vi "UG-DGXMLGen.vi"() -> ()   [LabVIEW 2012]
uses:
  <vilib>/xml/Load XML File.vi
  <vilib>/xml/Close Reference(Node).vi
  <resource>/objmgr/DOMUserDefRef.rc
  <vilib>/xml/NI_XML.lvlib
panel:
  out "error out":errorcluster
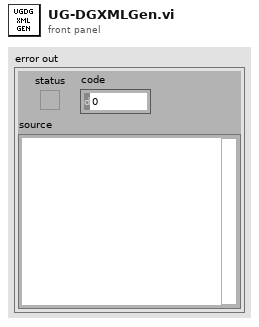
[diagram p1: front panel]
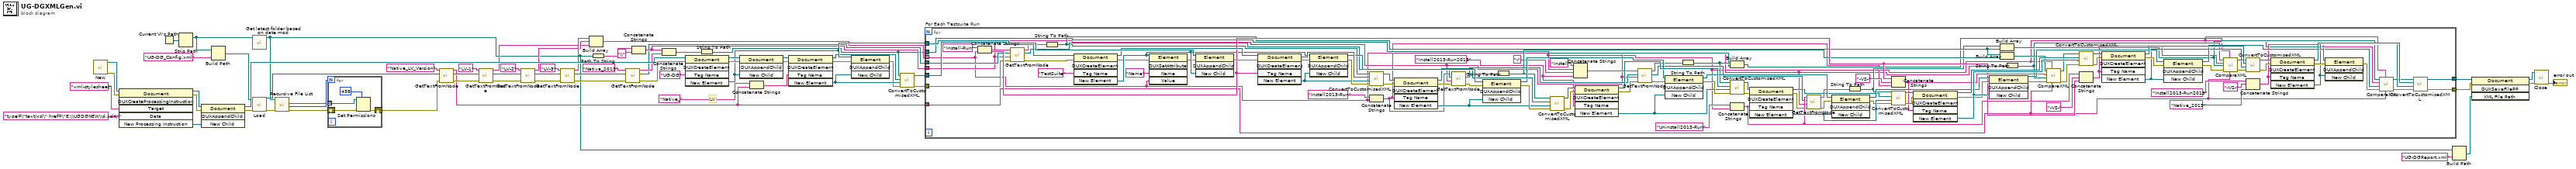
[diagram p0: block diagram]
diagram:
  # "LV"
  n1 = call <vilib>:"New.vi"() -> ("error out"=w59:errorcluster, "DOM document out"=w60:refnum<k20>)  [unwired: 1 in, 7 out]
  n2 = invoke class="Document" method="DUXCreateProcessingInstruction"(reference=w60, error in=w59, "Target"="xml-stylesheet" ("Value"), "Data"="type=\"text/xsl\" href=\"E:\\UGDGNEW\\d.xslt\"") -> (reference out=w65:refnum<k20>, error out=w64:errorcluster, "New Processing Instruction"=w63:refnum<k20>)  [unwired: 2 in, 3 out]
  n3 = Current VI's Path() -> (path=w8:path)
  n4 = Strip Path(path=w8) -> (stripped path=w7:path)  [unwired: 1 out]
  n5 = invoke class="Document" method="DUXAppendChild"(reference=w65, error in=w64, "New Child"=w63) -> (reference out=w58:refnum<k20>, error out=w27:errorcluster)  [unwired: 1 in, 2 out]
  n6 = Build Path(base path=w7, name or relative path="UG-DG_Config.xml") -> (appended path=w15:path)
  n7 = call "Get latest folder based on date mod.vi"("path"=w7) -> ("appended path"=w6:path)  [unwired: 10 in]
  n8 = call-poly <vilib>:"Load.vi"("path to XML document"=w15, "error in (no error)"=w27) -> ("DOM document out"=w42:refnum<k20>, "error out"=w2:errorcluster)  [unwired: 11 in, 1 out]
  n9 = call <vilib>:"Recursive File List.vi"("error in (no error)"=w2, "Folder Path"=w6) -> ("error out"=w3:errorcluster, "Number of Files"=w5:i32, "All Files in Dir"=w4:path[])  [unwired: 5 in, 2 out]
  n10 = for {
    N: w5 -> [_]
    tunnel: w4 -> [w71] mode=indexing
    shift-right: [w69] -> w1
    shift-left: w3 -> [w68]
    n11 = Set Permissions(7:i16 438 ("permissions"), 8:w68, 11:w71) -> (0:w69:errorcluster)  [unwired: 2 in, 1 out]
  }
  n12 = call "GetTextFromNode.vi"("error in (no error)"=w1, "node in"=w42, "Text"="Native_LV_Version" ("XPath expression")) -> ("error out"=w33:errorcluster, "node out"=w40:refnum<k20>, "Failure-db path"=w9:string)  [unwired: 6 in]
  n13 = call "GetTextFromNode.vi"("error in (no error)"=w33, "node in"=w40, "Text"="LV-1") -> ("error out"=w34:errorcluster, "node out"=w36:refnum<k20>, "Failure-db path"=w30:string)  [unwired: 6 in]
  n14 = call "GetTextFromNode.vi"("error in (no error)"=w34, "node in"=w36, "Text"="LV-2") -> ("error out"=w28:errorcluster, "node out"=w35:refnum<k20>, "Failure-db path"=w31:string)  [unwired: 6 in]
  n15 = call "GetTextFromNode.vi"("error in (no error)"=w28, "node in"=w35, "Text"="LV-3") -> ("error out"=w11:errorcluster, "node out"=w12:refnum<k20>, "Failure-db path"=w32:string)  [unwired: 6 in]
  n16 = Build Array(w32, w31, w30) -> (w29:string[])
  n17 = Path To String(path=w6) -> (string=w10:string)
  n18 = call "GetTextFromNode.vi"("error in (no error)"=w11, "node in"=w12, "Text"="Native_2013") -> ("error out"=w25:errorcluster, "node out"=w20:refnum<k20>, "Failure-db path"=w23:string)  [unwired: 6 in]
  n19 = Concatenate Strings(w10, "\\" ("string")) -> (w21:string)
  n20 = Concatenate Strings(w21, w23) -> (w22:string)
  n21 = invoke class="Document" method="DUXCreateElement"(reference=w58, error in=w25, "Tag Name"="UG-DG") -> (reference out=w66:refnum<k20>, error out=w57:errorcluster, "New Element"=w56:refnum<k20>)  [unwired: 2 in, 2 out]
  n22 = String To Path(string=w22) -> (path=w19:path)
  n23 = invoke class="Document" method="DUXAppendChild"(reference=w66, error in=w57, "New Child"=w56) -> (reference out=w54:refnum<k20>, error out=w55:errorcluster)  [unwired: 1 in, 2 out]
  n24 = Concatenate Strings("Native_" ("Tag Name"), w9) -> (w43:string)
  n25 = invoke class="Document" method="DUXCreateElement"(reference=w54, error in=w55, "Tag Name"=w43) -> (reference out=w51:refnum<k20>, error out=w53:errorcluster, "New Element"=w52:refnum<k20>)  [unwired: 2 in, 2 out]
  n26 = invoke class="Element" method="DUXAppendChild"(reference=w56, error in=w53, "New Child"=w52) -> (error out=w50:errorcluster)  [unwired: 1 in, 3 out]
  n27 = call "ConvertToCustomisedXML.vi"("error in"=w50, "New Element"=w52, "DOM document"=w51, "Path"=w19) -> ("error out"=w18:errorcluster, "DOM document out"=w17:refnum<k20>)  [unwired: 6 in]
  n28 = for "For Each Testsuite Run" {
    tunnel: w56 -> [w176]
    tunnel: w29 -> [w72] mode=indexing
    tunnel: [w118] -> w49
    tunnel: w17 -> [w177]
    tunnel: [w113] -> w45
    tunnel: w20 -> [w111]
    tunnel: w18 -> [w110]
    tunnel: w21 -> [w75]
    tunnel: w19 -> [w87]
    tunnel: w9 -> [w73]
    w76 = "Install2013-Run2013"
    n29 = Concatenate Strings("Install-Run", w72) -> (w112:string)
    n30 = call "GetTextFromNode.vi"("error in (no error)"=w110, "Failure db-folderpath"=w75, "node in"=w111, "Text"=w112) -> ("error out"=w109:errorcluster, "node out"=w106:refnum<k20>, "Failure-db path"=w103:string)  [unwired: 5 in]
    n31 = String To Path(string=w103) -> (path=w91:path)
    n32 = invoke class="Document" method="DUXCreateElement"(reference=w177, error in=w109, "Tag Name"="TestSuite") -> (reference out=w174:refnum<k20>, error out=w82:errorcluster, "New Element"=w83:refnum<k20>)  [unwired: 2 in, 2 out]
    n33 = invoke class="Element" method="DUXSetAttribute"(reference=w83, error in=w82, "Name"="Name", "Value"=w72) -> (error out=w81:errorcluster)  [unwired: 1 in, 4 out]
    n34 = invoke class="Element" method="DUXAppendChild"(reference=w176, error in=w81, "New Child"=w83) -> (error out=w122:errorcluster)  [unwired: 1 in, 3 out]
    n35 = invoke class="Document" method="DUXCreateElement"(reference=w174, error in=w122, "Tag Name"=w112) -> (reference out=w173:refnum<k20>, error out=w171:errorcluster, "New Element"=w155:refnum<k20>)  [unwired: 2 in, 2 out]
    n36 = invoke class="Element" method="DUXAppendChild"(reference=w83, error in=w171, "New Child"=w155) -> (reference out=w167:refnum<k20>, error out=w172:errorcluster)  [unwired: 1 in, 2 out]
    n37 = call "ConvertToCustomisedXML.vi"("error in"=w172, "New Element"=w155, "DOM document"=w173, "Path"=w91) -> ("error out"=w168:errorcluster, "DOM document out"=w169:refnum<k20>)  [unwired: 6 in]
    n38 = Concatenate Strings("Install2013-Run", w72) -> (w85:string)
    n39 = invoke class="Document" method="DUXCreateElement"(reference=w169, error in=w168, "Tag Name"=w85) -> (reference out=w166:refnum<k20>, error out=w108:errorcluster, "New Element"=w154:refnum<k20>)  [unwired: 2 in, 2 out]
    n40 = call "GetTextFromNode.vi"("error in (no error)"=w108, "Failure db-folderpath"=w75, "node in"=w106, "Text"=w85) -> ("error out"=w107:errorcluster, "node out"=w104:refnum<k20>, "Failure-db path"=w102:string)  [unwired: 5 in]
    n41 = invoke class="Element" method="DUXAppendChild"(reference=w167, error in=w107, "New Child"=w154) -> (reference out=w161:refnum<k20>, error out=w165:errorcluster)  [unwired: 1 in, 2 out]
    n42 = String To Path(string=w102) -> (path=w93:path)
    n43 = call "ConvertToCustomisedXML.vi"("error in"=w165, "New Element"=w154, "DOM document"=w166, "Path"=w93) -> ("error out"=w163:errorcluster, "DOM document out"=w164:refnum<k20>)  [unwired: 6 in]
    n44 = Concatenate Strings("Install" ("element"), w72, "-" ("string"), w76) -> (w78:string)
    n45 = invoke class="Document" method="DUXCreateElement"(reference=w164, error in=w163, "Tag Name"=w76) -> (reference out=w162:refnum<k20>, error out=w105:errorcluster, "New Element"=w153:refnum<k20>)  [unwired: 2 in, 2 out]
    n46 = call "GetTextFromNode.vi"("error in (no error)"=w105, "Failure db-folderpath"=w75, "node in"=w104, "Text"=w78) -> ("error out"=w100:errorcluster, "node out"=w98:refnum<k20>, "Failure-db path"=w101:string)  [unwired: 5 in]
    n47 = invoke class="Element" method="DUXAppendChild"(reference=w161, error in=w100, "New Child"=w153) -> (reference out=w146:refnum<k20>, error out=w160:errorcluster)  [unwired: 1 in, 2 out]
    n48 = String To Path(string=w101) -> (path=w88:path)
    n49 = Build Array(w88, w87) -> (w86:path[])
    n50 = call "ConvertToCustomisedXML.vi"("error in"=w160, "New Element"=w153, "DOM document"=w162, "Path"=w88) -> ("error out"=w156:errorcluster, "DOM document out"=w159:refnum<k20>)  [unwired: 6 in]
    n51 = Concatenate Strings("Uninstall2013-Run" ("Tag Name"), w72) -> (w99:string)
    n52 = invoke class="Document" method="DUXCreateElement"(reference=w159, error in=w156, "Tag Name"=w99) -> (reference out=w94:refnum<k20>, error out=w97:errorcluster, "New Element"=w158:refnum<k20>)  [unwired: 2 in, 2 out]
    n53 = call "GetTextFromNode.vi"("error in (no error)"=w97, "Failure db-folderpath"=w75, "node in"=w98, "Text"=w99) -> ("error out"=w96:errorcluster, "Failure-db path"=w95:string)  [unwired: 5 in, 1 out]
    n54 = invoke class="Element" method="DUXAppendChild"(reference=w146, error in=w96, "New Child"=w158) -> (reference out=w145:refnum<k20>, error out=w157:errorcluster)  [unwired: 1 in, 2 out]
    n55 = String To Path(string=w95) -> (path=w90:path)
    n56 = Concatenate Strings(w112, "-VS-" ("string"), w85) -> (w117:string)
    n57 = call "ConvertToCustomisedXML.vi"("error in"=w157, "New Element"=w158, "DOM document"=w94, "Path"=w90) -> ("error out"=w135:errorcluster, "DOM document out"=w148:refnum<k20>)  [unwired: 6 in]
    n58 = invoke class="Document" method="DUXCreateElement"(reference=w148, error in=w135, "Tag Name"=w117) -> (reference out=w150:refnum<k20>, error out=w149:errorcluster, "New Element"=w151:refnum<k20>)  [unwired: 2 in, 2 out]
    n59 = invoke class="Element" method="DUXAppendChild"(reference=w145, error in=w149, "New Child"=w151) -> (reference out=w136:refnum<k20>, error out=w144:errorcluster)  [unwired: 1 in, 2 out]
    n60 = Build Array(w90, w91) -> (w89:path[])
    n61 = Build Array(w91, w93) -> (w92:path[])
    n62 = String To Path(string=w75) -> (path=w74:path)
    n63 = call "CompareXML.vi"("Native LV Version"=w73, "Lv Version"=w72, "error in"=w144, "file path (use dialog)"=w74, "name or relative path"=w117, "Failure_DB__File_Paths_Array"=w92) -> ("error out"=w143:errorcluster, "XML File Path(duplicate)"=w121:path)  [unwired: 4 in]
    n64 = call "ConvertToCustomisedXML.vi"("error in"=w143, "New Element"=w151, "DOM document"=w150, "Path"=w121) -> ("error out"=w137:errorcluster, "DOM document out"=w138:refnum<k20>)  [unwired: 6 in]
    n65 = Concatenate Strings(w99, "-VS-" ("string"), w112) -> (w116:string)
    n66 = invoke class="Document" method="DUXCreateElement"(reference=w138, error in=w137, "Tag Name"=w116) -> (reference out=w142:refnum<k20>, error out=w141:errorcluster, "New Element"=w115:refnum<k20>)  [unwired: 2 in, 2 out]
    n67 = invoke class="Element" method="DUXAppendChild"(reference=w136, error in=w141, "New Child"=w115) -> (reference out=w128:refnum<k20>, error out=w140:errorcluster)  [unwired: 1 in, 2 out]
    n68 = call "CompareXML.vi"("Native LV Version"=w73, "Lv Version"=w72, "error in"=w140, "file path (use dialog)"=w74, "name or relative path"=w116, "Failure_DB__File_Paths_Array"=w89) -> ("error out"=w139:errorcluster, "XML File Path(duplicate)"=w120:path)  [unwired: 4 in]
    n69 = call "ConvertToCustomisedXML.vi"("error in"=w139, "New Element"=w115, "DOM document"=w142, "Path"=w120) -> ("error out"=w124:errorcluster, "DOM document out"=w129:refnum<k20>)  [unwired: 6 in]
    n70 = Concatenate Strings("Install2013-Run2013" ("string"), "-VS-" ("string"), "Native_2013" ("string")) -> (w114:string)
    n71 = invoke class="Document" method="DUXCreateElement"(reference=w129, error in=w124, "Tag Name"=w114) -> (reference out=w133:refnum<k20>, error out=w132:errorcluster, "New Element"=w123:refnum<k20>)  [unwired: 2 in, 2 out]
    n72 = invoke class="Element" method="DUXAppendChild"(reference=w128, error in=w132, "New Child"=w123) -> (error out=w131:errorcluster)  [unwired: 1 in, 3 out]
    n73 = call "CompareXML.vi"("Native LV Version"=w73, "Lv Version"=w72, "error in"=w131, "file path (use dialog)"=w74, "name or relative path"=w114, "Failure_DB__File_Paths_Array"=w86) -> ("error out"=w130:errorcluster, "XML File Path(duplicate)"=w119:path)  [unwired: 4 in]
    n74 = call "ConvertToCustomisedXML.vi"("error in"=w130, "New Element"=w123, "DOM document"=w133, "Path"=w119) -> ("error out"=w118:errorcluster, "DOM document out"=w113:refnum<k20>)  [unwired: 6 in]
  }
  n75 = Build Path(base path=w6, name or relative path="UG-DGReport.xml") -> (appended path=w13:path)
  n76 = invoke class="Document" method="DUXSaveFilePP"(reference=w45, error in=w49, "XML File Path"=w13) -> (reference out=w48:refnum<k20>, error out=w47:errorcluster)  [unwired: 1 in, 2 out]
  n77 = call-poly <vilib>:"Close.vi"("error in (no error)"=w47, "node"=w48) -> ("error out"=→"error out":errorcluster)  [unwired: 7 in]
